vi "Drive Controller.vi"(8 "error in":errorcluster) -> ()   [LabVIEW 2020]
doc: "This VI executes continuously carrying out the current operation and responding to updates or new operation requests. It will often contain the timing or control code that is difficult to place directly in TeleOp. This VI generally opens all sensors and motors and isolates the rest of the robot code from knowing implementation details of how the operations are carried out."
uses:
  <vilib>/Rock Robotics/WPI/Framework/Completion Status.ctl
  Drive Setpoints.ctl
  Drive Operations.ctl
  <vilib>/Rock Robotics/WPI/SafetyOutput/WPI_SafetyOutputConfigMenu.ctl
  <vilib>/Rock Robotics/WPI/RobotDrive/WPI_RobotDriveOpen2MotorWithExistingMotors.vi
  <vilib>/Rock Robotics/Network Tables/NT Write Numeric Array.vi
panel:
  in  "Interactive Values":T1
  in  "Buttons":cluster{"Execute Cmd":bool, "Abort Cmd":bool}
  out "Command Timing":cluster{"Start Time (ms)":u32, "Iterations":i32}
  out "Status":T3
  out "Setpoints":T4(graph)
  out "Current\nCmd":string
  # "Tip: The graph shows the motor setpoints. It may also be helpful to observe inputs and sensor values.\nYou may also want to display tuning or debugging controls."
  # "Interactive Command: You may fill in the settings for a command\nand schedule it with the Execute button. You can observe and abort\nany command while fine tuning the code for the controller."
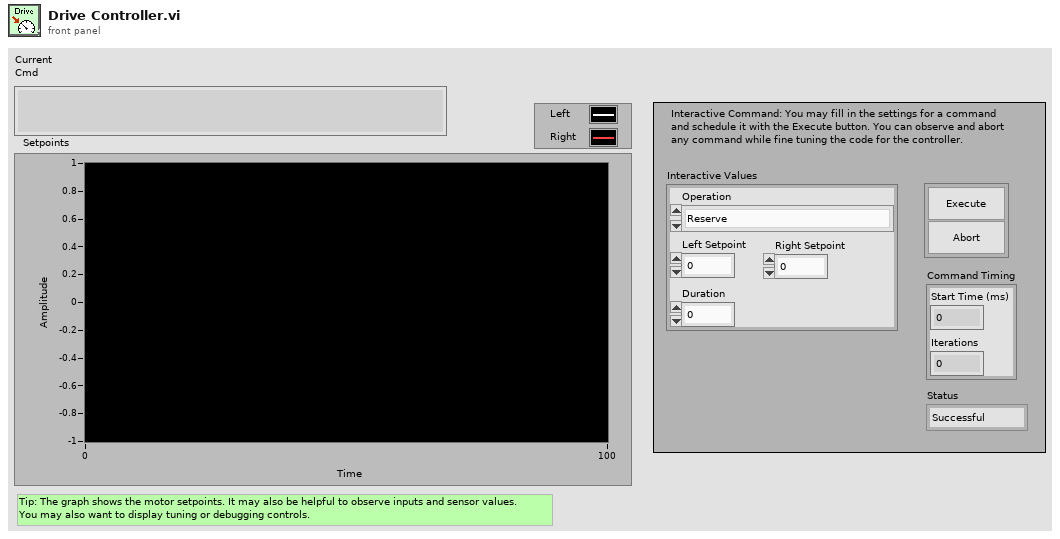
[diagram p1: front panel]
types:
  T1 = typedef "Drive Setpoints.ctl" = cluster{"Operation":T2, "Left Setpoint":dbl, "Right Setpoint":dbl, "Duration":dbl}
  T2 = typedef "Drive Operations.ctl" = enum16{"Reserve", "Read Current", "Immediate", "Drive for Time", "Drive for Distance"}
  T3 = typedef "Completion Status.ctl" = enum16{"Successful", "Aborted", "Incomplete"}
  T4 = cluster{"Left Setpoint":dbl, "Right Setpoint":dbl}
  T5 = typedef "WPI_SafetyOutputConfigMenu.ctl" = enum16{"Enable", "Disable"}
  T6 = typedef "WPI_MotorControlDeviceRef.ctl" = cluster{"DeviceStatus":errorcluster, "Type":T7, "PWM":cluster{"PWM Channel":T8, "DeadBand":T9}, "CAN":cluster{"Device Number":u8, "SetOutput VI Ref":variant, "GetOutput VI Ref":variant, "Enable VI Ref":variant, "Disable VI Ref":variant, "Data":variant}, "Invert":bool, "DIO PWM":cluster{"PWM \"Enable\" Channel":T8, "DIOChannel":T10, "PWM Rate":dbl}}
  T7 = typedef "WPI_MotorControlType.ctl" = enum16{"PWM", "CAN", "DIO PWM"}
  T8 = typedef "FPGA_DIOPWMChannel.ctl" = enum8{"PWM 0", "PWM 1", "PWM 2", "PWM 3", "PWM 4", "PWM 5", "PWM 6", "PWM 7", "PWM 8", "PWM 9", "PWM MXP 0", "PWM MXP 1", "PWM MXP 2", "PWM MXP 3", "PWM MXP 4", "PWM MXP 5", "PWM MXP 6", "PWM MXP 7", "PWM MXP 8", "PWM MXP 9", "Invalid"}
  T9 = typedef "WPI_PWMDeadband.ctl" = cluster{"Name":string, "maxPositivePwm":i32, "minPositivePwm":i32, "centerPwm":i32, "maxNegativePwm":i32, "minNegativePwm":i32, "angularRange":u16}
  T10 = typedef "FPGA_DIOChannel.ctl" = enum8{"DIO 0", "DIO 1", "DIO 2", "DIO 3", "DIO 4", "DIO 5", "DIO 6", "DIO 7", "DIO 8", "DIO 9", "DIO MXP 0", "DIO MXP 1", "DIO MXP 2", "DIO MXP 3", "DIO MXP 4", "DIO MXP 5", "DIO MXP 6", "DIO MXP 7", "DIO MXP 8", "DIO MXP 9", "DIO MXP 10", "DIO MXP 11", "DIO MXP 12", "DIO MXP 13", "DIO MXP 14", "DIO MXP 15", "SPI Port CS1", "SPI Port CS2", "SPI Port CS3", "SPI Port MISO", "SPI Port MOSI", "Invalid"}
  T11 = typedef "WPI_RobotDriveDevRef.ctl" = cluster{"DevStatus":errorcluster, "Motors[]":T6[], "Square Inputs":bool, "Max Output":dbl}
  T12 = typedef "Command Status Info.ctl" = cluster{"Name":string, "Status":T3, "notifier out":T13}
  T13 = typedef "Completion Notifier.ctl" = refnum<notifier>
  T14 = cluster{"SubSystem Data":T1, cluster{"Start Time (ms)":u32, "Iterations":i32}, cluster{"Command Info":T12, "Description":string, "Default Command":T1, "queue out":refnum<queue>, "Subsystem Name":string}}
  T15 = cluster{"SubSystem Data":T1, cluster{"Start Time (ms)":u32, "Iterations":i32}, "Default Command Arguments":cluster{"Command Info":T12, "Description":string, "Default Command":T1, "queue out":refnum<queue>, "Subsystem Name":string}}
  T16 = cluster{"Don't move motors while reserved":dbl, "Don't move motors while reserved":dbl}
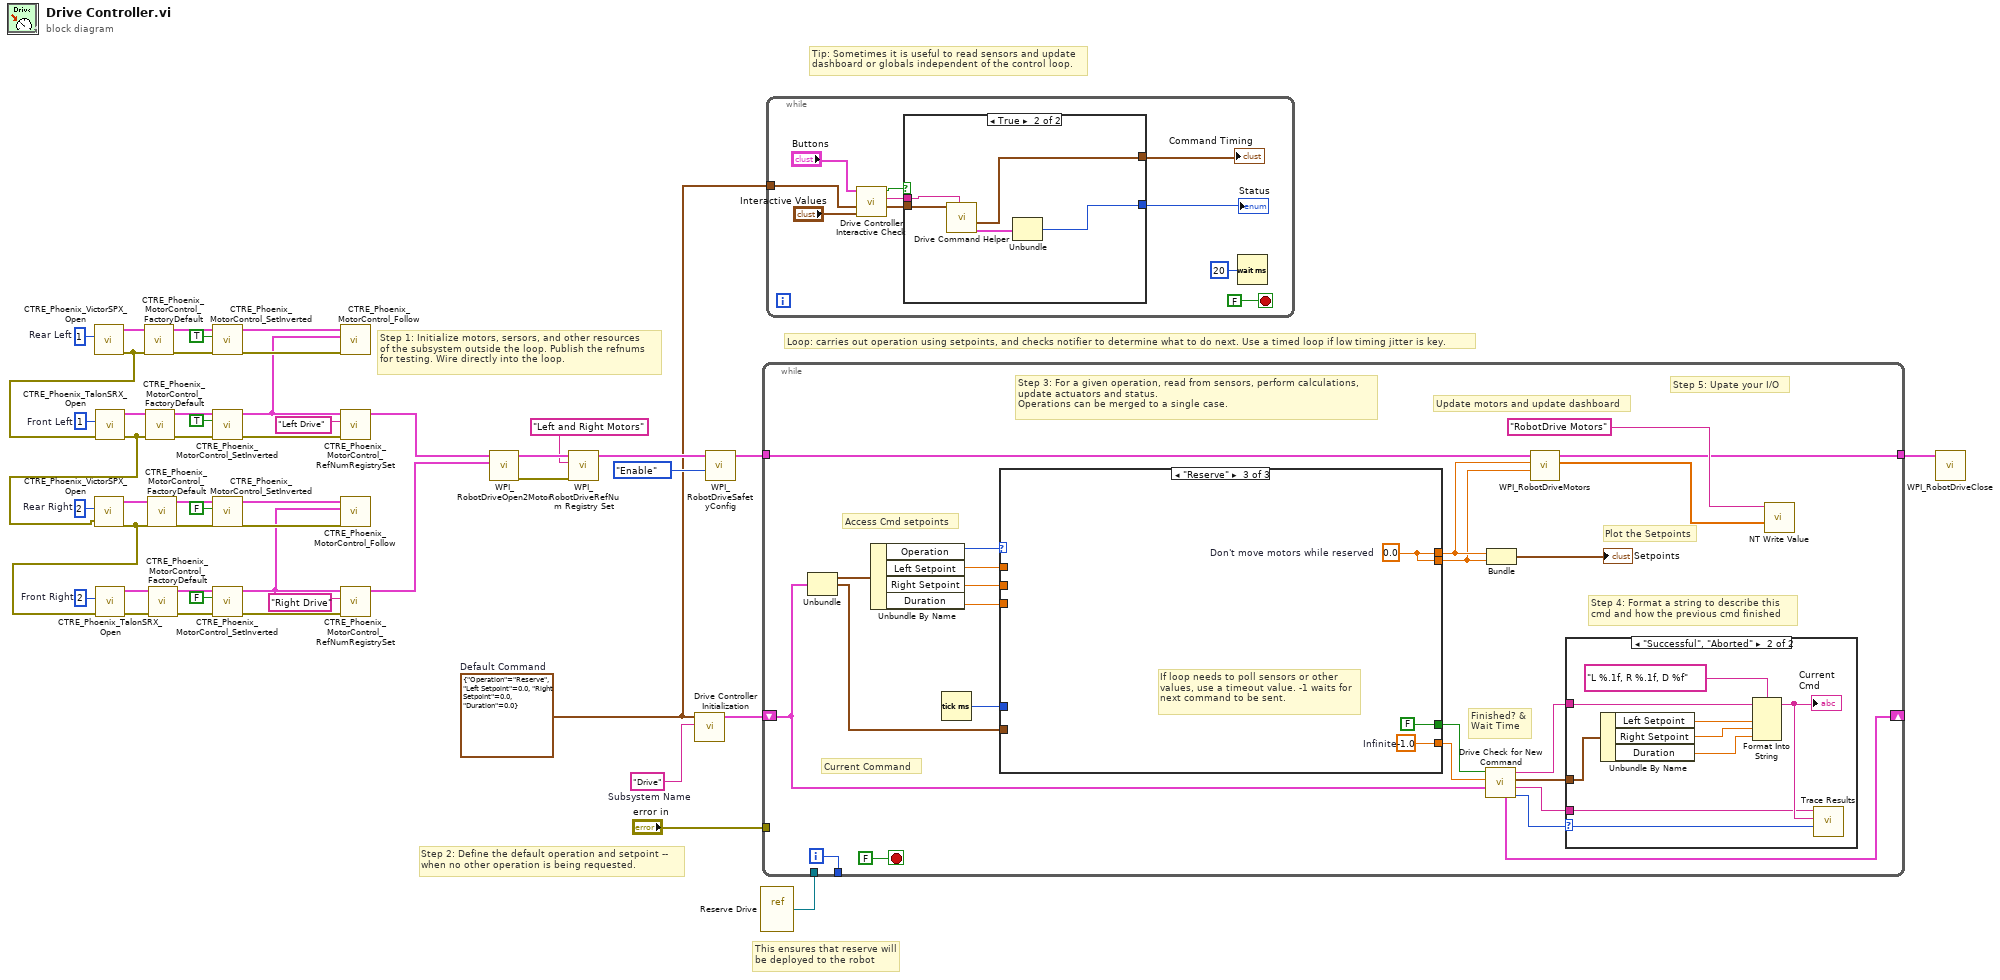
[diagram p0: block diagram]
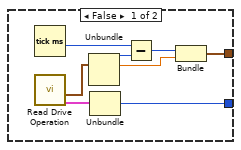
[diagram p2: hidden frame]
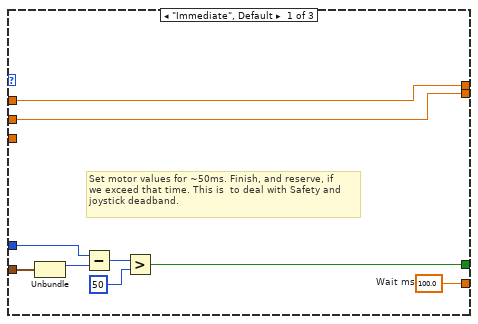
[diagram p4: hidden frame]
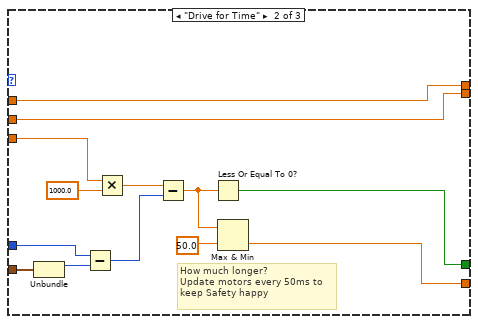
[diagram p5: hidden frame]
diagram:
  w7 = u8 2  # Front Right
  w8 = u8 2  # Rear Right
  w9 = u8 1  # Front Left
  w10 = u8 1  # Rear Left
  w38 = T1 {"Operation"=enum."Reserve", "Left Setpoint"=0.0, "Right Setpoint"=0.0, "Duration"=0.0}  # Default Command
  w48 = "Drive"  # Subsystem Name
  # "This ensures that reserve will\nbe deployed to the robot"
  # "Tip: Sometimes it is useful to read sensors and update\ndashboard or globals independent of the control loop."
  # "Step 2: Define the default operation and setpoint --\nwhen no other operation is being requested."
  # "Step 1: Initialize motors, sersors, and other resources\nof the subsystem outside the loop. Publish the refnums\nfor testing. Wire directly into the loop."
  # "Loop: carries out operation using setpoints, and checks notifier to determine what to do next. Use a timed loop if low timing jitter is key."
  n1 = call <vilib>:"CTRE_Phoenix_VictorSPX_Open.vi"("Device Number"=w10) -> ("error out"=w3:errorcluster, "PhoenixMotorControlDevRef"=w37:T6)  [unwired: 9 in]
  n2 = call <vilib>:"CTRE_Phoenix_TalonSRX_Open.vi"("error in"=w3, "Device Number"=w9) -> ("error out"=w2:errorcluster, "PhoenixMotorControlDevRef"=w31:T6)  [unwired: 8 in]
  n3 = call <vilib>:"CTRE_Phoenix_VictorSPX_Open.vi"("error in"=w2, "Device Number"=w8) -> ("error out"=w1:errorcluster, "PhoenixMotorControlDevRef"=w36:T6)  [unwired: 8 in]
  n4 = call <vilib>:"CTRE_Phoenix_TalonSRX_Open.vi"("error in"=w1, "Device Number"=w7) -> ("error out"=w30:errorcluster, "PhoenixMotorControlDevRef"=w29:T6)  [unwired: 8 in]
  n5 = call <vilib>:"CTRE_Phoenix_MotorControl_FactoryDefault.vi"("error in"=w3, "PhoenixMotorControlDevRef"=w37) -> ("error out"=w33:errorcluster, "PhoenixMotorControlDevRef"=w32:T6)  [unwired: 8 in]
  n6 = call <vilib>:"CTRE_Phoenix_MotorControl_FactoryDefault.vi"("error in"=w2, "PhoenixMotorControlDevRef"=w31) -> ("error out"=w26:errorcluster, "PhoenixMotorControlDevRef"=w25:T6)  [unwired: 8 in]
  n7 = call <vilib>:"CTRE_Phoenix_MotorControl_FactoryDefault.vi"("error in"=w1, "PhoenixMotorControlDevRef"=w36) -> ("error out"=w35:errorcluster, "PhoenixMotorControlDevRef"=w34:T6)  [unwired: 8 in]
  n8 = call <vilib>:"CTRE_Phoenix_MotorControl_FactoryDefault.vi"("error in"=w30, "PhoenixMotorControlDevRef"=w29) -> ("error out"=w28:errorcluster, "PhoenixMotorControlDevRef"=w27:T6)  [unwired: 8 in]
  n9 = call <vilib>:"CTRE_Phoenix_MotorControl_SetInverted.vi"("error in (no error)"=w33, "Invert?"=TRUE, "PhoenixMotorControlDevRef"=w32) -> ("error out"=w22:errorcluster, "PhoenixMotorControlDevRef"=w21:T6)  [unwired: 7 in]
  n10 = call <vilib>:"CTRE_Phoenix_MotorControl_SetInverted.vi"("error in (no error)"=w26, "Invert?"=TRUE, "PhoenixMotorControlDevRef"=w25) -> ("error out"=w24:errorcluster, "PhoenixMotorControlDevRef"=w14:T6)  [unwired: 7 in]
  n11 = call <vilib>:"CTRE_Phoenix_MotorControl_SetInverted.vi"("error in (no error)"=w35, "Invert?"=FALSE, "PhoenixMotorControlDevRef"=w34) -> ("error out"=w20:errorcluster, "PhoenixMotorControlDevRef"=w19:T6)  [unwired: 7 in]
  n12 = call <vilib>:"CTRE_Phoenix_MotorControl_SetInverted.vi"("error in (no error)"=w28, "Invert?"=FALSE, "PhoenixMotorControlDevRef"=w27) -> ("error out"=w23:errorcluster, "PhoenixMotorControlDevRef"=w13:T6)  [unwired: 7 in]
  n13 = call <vilib>:"CTRE_Phoenix_MotorControl_Follow.vi"("error in (no error)"=w22, "Master Controller to Follow"=w14, "PhoenixMotorControlDevRef"=w21) -> ()  [unwired: 7 in, 2 out]
  n14 = call <vilib>:"CTRE_Phoenix_MotorControl_RefNumRegistrySet.vi"("error in (no error)"=w24, "refnum name"="Left Drive", "PhoenixMotorControlDevRef"=w14) -> ("PhoenixMotorControlDevRef"=w6:T6)  [unwired: 7 in, 1 out]
  n15 = call <vilib>:"CTRE_Phoenix_MotorControl_Follow.vi"("error in (no error)"=w20, "Master Controller to Follow"=w13, "PhoenixMotorControlDevRef"=w19) -> ()  [unwired: 7 in, 2 out]
  n16 = call <vilib>:"CTRE_Phoenix_MotorControl_RefNumRegistrySet.vi"("error in (no error)"=w23, "refnum name"="Right Drive", "PhoenixMotorControlDevRef"=w13) -> ("PhoenixMotorControlDevRef"=w5:T6)  [unwired: 7 in, 1 out]
  n17 = call-poly <vilib>:"WPI_RobotDriveOpen2Motor.vi"("Right Motor Dev Ref"=w5, "Left Motor Dev Ref"=w6) -> ("error out"=w45:errorcluster, "RobotDriveDevRef"=w47:T11)  [unwired: 3 in, 5 out]
  n18 = call <vilib>:"WPI_RobotDriveRefNum Registry Set.vi"("error in (no error)"=w45, "refnum name"="Left and Right Motors", "RobotDriveDevRef"=w47) -> ("RobotDriveDevRef"=w44:T11)  [unwired: 1 in, 7 out]
  n19 = call "Drive Controller Initialization.vi"("Subsystem Name"=w48, "Default Command"=w38) -> ("Current Command"=w40:T14)  [unwired: 9 in]
  n20 = call <vilib>:"WPI_RobotDriveSafetyConfig.vi"("mode"=WPI_SafetyOutputConfigMenu."Enable", "RobotDriveDevRef"=w44) -> ("RobotDriveDevRef"=w42:T11)  [unwired: 8 in, 1 out]
  n21 = vi-ref "Reserve Drive.vi"() -> (w39:refnum<vi>)
  n22 = while {
    shift-right: [w59] -> _
    shift-left: w40 -> [w52]
    tunnel: [w71] -> _
    tunnel: w42 -> [w67]
    tunnel: "error in" -> [_]
    tunnel: w39 -> [_]
    tunnel: [w49] -> w4
    i -> [w71]
    stop <- FALSE stop-if-true
    # "Step 5: Upate your I/O"
    # "Step 4: Format a string to describe this\ncmd and how the previous cmd finished"
    # "Current Command"
    # "Update motors and update dashboard"
    # "Plot the Setpoints"
    # "Access Cmd setpoints"
    # "Finished? &\nWait Time"
    # "Step 3: For a given operation, read from sensors, perform calculations,\nupdate actuators and status.\nOperations can be merged to a single case."
    n23 = Unbundle(w52) -> ("SubSystem Data"=w66:T1, w53:cluster{"Start Time (ms)":u32, "Iterations":i32})  [unwired: 1 out]
    n24 = Unbundle By Name(w66) -> ("Operation"=w65:T2, "Left Setpoint"=w64:dbl, "Right Setpoint"=w63:dbl, "Duration"=w62:dbl)
    n25 = Tick Count (ms)() -> (millisecond timer value=w61:u32)
    n26 = case shown="\"Reserve\"" w65 {
      tunnel: [w90 w91 w106] -> w58
      tunnel: [w83 w98 FALSE ("ignore previous (F)")] -> w57
      tunnel: w53 -> [w82 w100 _]
      tunnel: [w89 w97 w104] -> w69
      tunnel: [w88 w96 w104] -> w68
      tunnel: w64 -> [w89 w97 _]
      tunnel: w63 -> [w88 w96 _]
      tunnel: w62 -> [_ w95 _]
      tunnel: w61 -> [w84 w94 _]
      frame "Immediate", Default {
        w90 = 100.0  # Wait ms
        # "Set motor values for ~50ms. Finish, and reserve, if\nwe exceed that time. This is  to deal with Safety and\njoystick deadband."
        n27 = Unbundle(w82) -> ("Start Time (ms)"=w85:u32)  [unwired: 1 out]
        n28 = Subtract(x=w84, y=w85) -> (x-y=w86:u32)
        n29 = Greater?(x=w86, y=u8 50 ("Left Motor")) -> (0:w83:bool)
      }
      frame "Drive for Time" {
        # "How much longer?\nUpdate motors every 50ms to\nkeep Safety happy"
        n30 = Unbundle(w100) -> ("Start Time (ms)"=w99:u32)  [unwired: 1 out]
        n31 = Subtract(x=w94, y=w99) -> (x-y=w103:u32)
        n32 = Multiply(x=w95, y=1000.0) -> (x*y=w102:dbl)
        n33 = Subtract(x=w102, y=w103) -> (x-y=w93:dbl)
        n34 = Less Or Equal To 0?(x=w93) -> (x <= 0?=w98:bool)
        n35 = Max & Min(x=w93, y=50.0) -> (min(x,y)=w91:dbl)  [unwired: 1 out]
      }
      frame "Reserve" {
        w104 = 0.0  # Don't move motors while reserved
        w106 = -1.0  # Infinite
        # "If loop needs to poll sensors or other\nvalues, use a timeout value. -1 waits for\nnext command to be sent."
      }
    }
    n36 = call "Drive Check for New Command.vi"("input cluster"=w52, "Wait time (ms)"=w58, "Finished?"=w57) -> ("Completion"=w60:T3, "Subsystem Name"=w54:string, "Current Command"=w55:T1, "Initial Trace String"=w56:string, "Next Command"=w59:T15)  [unwired: 4 in]
    n37 = Bundle("Don't move motors while reserved"=w69, "Don't move motors while reserved"=w68) -> (→"Setpoints":T16)  [unwired: 1 in]
    n38 = call <vilib>:"WPI_RobotDriveMotors.vi"("RightSpeed"=w68, "LeftSpeed"=w69, "RobotDriveDevRef"=w67) -> ("Motor Values"=w50:dbl[], "RobotDriveDevRef"=w49:T11)  [unwired: 1 in, 6 out]
    n39 = case shown="\"Successful\", \"Aborted\"" w60 {
      selector: w60 -> [_ w81]
      tunnel: w56 -> [_ w76]
      tunnel: w55 -> [_ w77]
      tunnel: w54 -> [_ w73]
      frame "Incomplete", Default {
        # "Continuing current command"
      }
      frame "Successful", "Aborted" {
        # "Report and setup for next command"
        n40 = Unbundle By Name(w77) -> ("Left Setpoint"=w79:dbl, "Right Setpoint"=w80:dbl, "Duration"=w74:dbl)
        n41 = Format Into String(format string="L %.1f, R %.1f, D %f", initial string=w76, w79, w80, w74) -> (resulting string=w75:string)  [unwired: 1 in, 1 out]
        "Current\nCmd" <- w75
        n42 = call <vilib>:"Trace Results.vi"("Status of previous command"=w81, "Description"=w75, "Subsystem"=w73) -> ()  [unwired: 9 in]
      }
    }
    n43 = call-poly <vilib>:"NT Write Value.vi"("Numeric Array"=w50, "Name"="RobotDrive Motors") -> ()  [unwired: 9 in, 1 out]
  }
  n44 = while {
    tunnel: w38 -> [w108]
    stop <- FALSE stop-if-true
    n45 = call "Drive Controller Interactive Check.vi"("Interactive Command In"="Interactive Values", "Default Command"=w108, "Buttons"="Buttons") -> ("Interactive Command Out"=w110:T1, "Trace String"=w111:string, "Schedule"=w112:bool)  [unwired: 6 in]
    n46 = case shown="True" w112 {
      tunnel: [w121 w129] -> w113
      tunnel: [w120 w125] -> w114
      tunnel: w111 -> [_ w127]
      tunnel: w110 -> [_ w126]
      frame False {
        n47 = Tick Count (ms)() -> (millisecond timer value=w124:u32)
        n48 = call "Read Drive Operation.vi"() -> ("Command Info"=w118:T12, "SubSystem Data"=w117:T1)  [unwired: 9 in, 1 out]
        n49 = Unbundle(w117) -> ("Operation"=w122:T2, "Left Setpoint"=w119:dbl)  [unwired: 2 out]
        n50 = Unbundle(w118) -> ("Status"=w121:T3)  [unwired: 2 out]
        n51 = Subtract(x=w124, y=w122) -> (x-y=w123:u32)
        n52 = Bundle(w123, "Left Setpoint"=w119) -> (w120:cluster{u32, "Left Setpoint":dbl})  [unwired: 1 in]
      }
      frame True {
        n53 = call "Drive Command Helper.vi"("Description"=w127, "SubSystem Data"=w126) -> ("Command Info Out"=w128:T12, "Command Timing"=w125:cluster{"Start Time (ms)":u32, "Iterations":i32})  [unwired: 7 in, 1 out]
        n54 = Unbundle(w128) -> ("Status"=w129:T3)  [unwired: 2 out]
      }
    }
    "Status" <- w113
    "Command Timing" <- w114
    n55 = Wait (ms)(milliseconds to wait=u32 20) -> ()  [unwired: 1 out]
  }
  n56 = call <vilib>:"WPI_RobotDriveClose.vi"("RobotDriveDevRef"=w4) -> ()  [unwired: 10 in, 1 out]
